vi "NI_9252 DataCollection.vi"(11 "device name":tag="cDAQ9189-21D2231Mod8") -> (3 "First Channel 1D data array":dbl[](array[numeric]))   [LabVIEW 2022 SP3]
uses:
  <vilib>/Analysis/baseanly.llb/Mean (DBL).vi
  STOP_GLOBAL.vi
  <vilib>/Analysis/NI_AALBase.lvlib
panel:
  out "Voltage Chamber Pressure  2":dynamicdata(graph)
  in  "Types of Testing":T1(tab)
  in  "Channel Array":dbl[](array[knob]) scale=0.0..10.0
  in  "maximum voltage":dbl=5.0 format="%0.2f"
  in  "minimum voltage":dbl=-5.0 format="%0.2f"
  in  "Output Channels":tag
  out "Mass Flow":dbl[](graph)
  out "Mass Flow":dynamicdata(graph)
  out "Chamber Pressure":dbl[](graph)
  out "Supply Pressure":dbl[](graph)
  out "Voltage Chamber Pressure":dynamicdata(graph)
  out "Voltage Supply Pressure":dynamicdata(graph)
  # "ANALOG VOLTAGE OUTPUT"
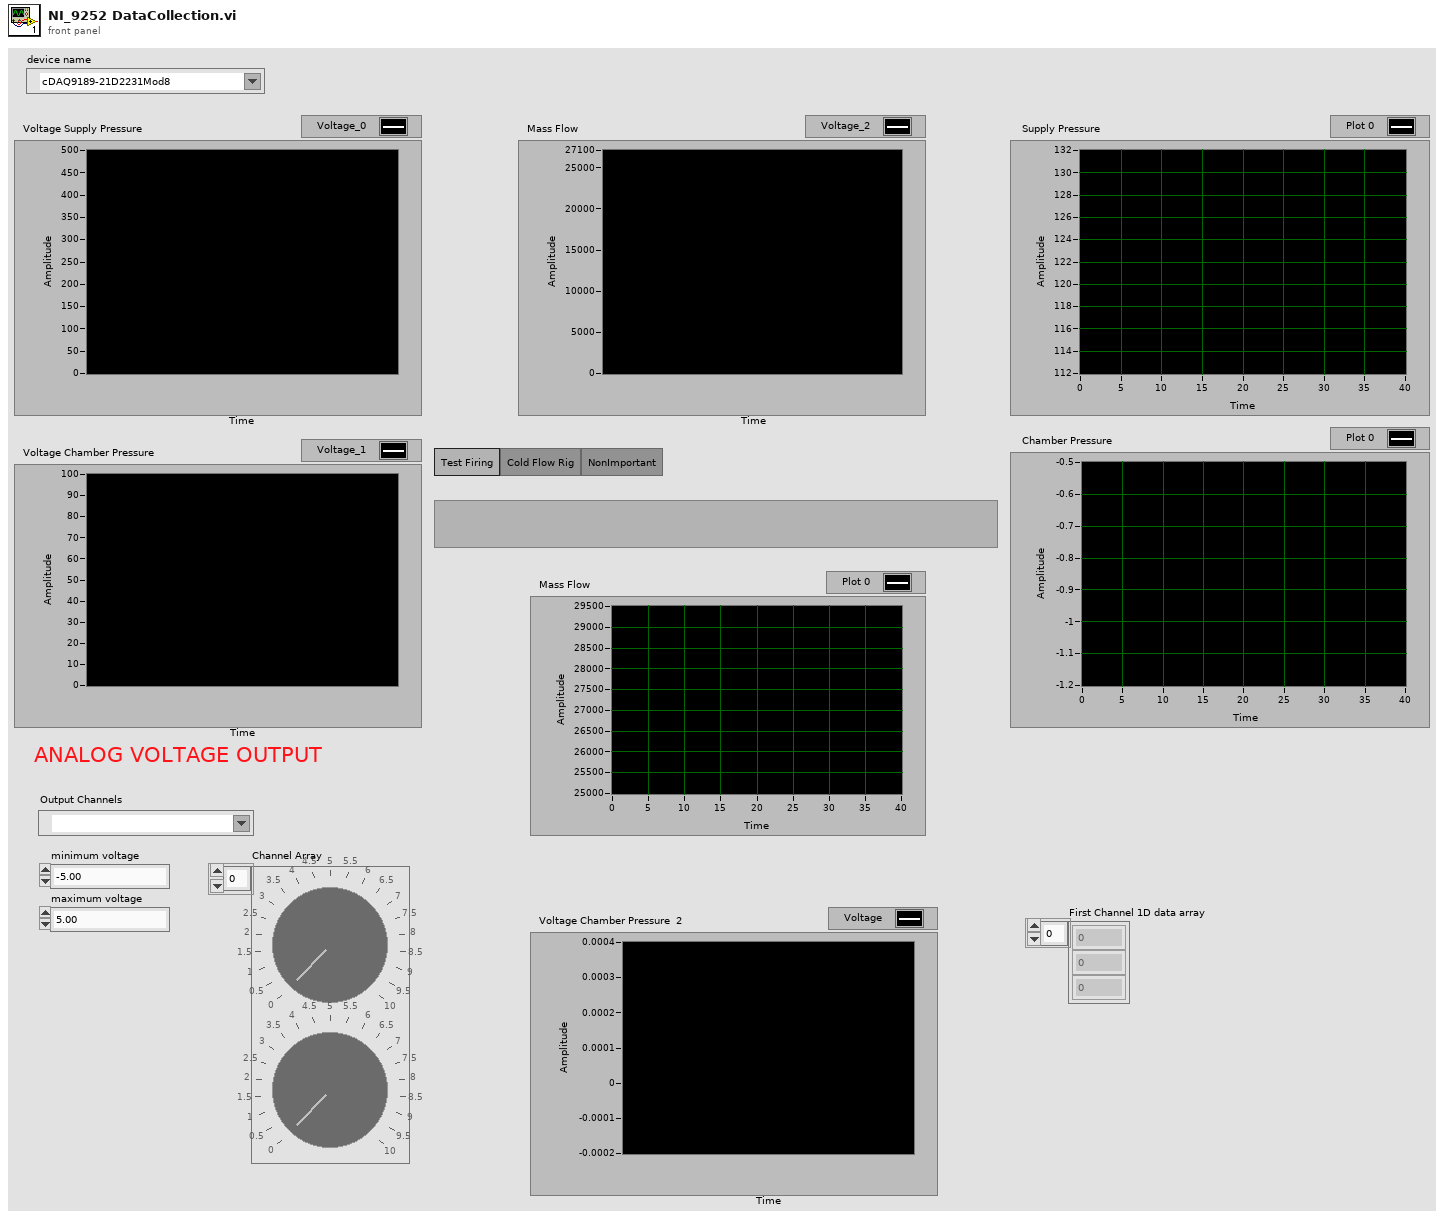
[diagram p1: front panel]
types:
  T1 = enum32{"Test Firing", "Cold Flow Rig", "NonImportant"}
  T2 = enum16{"Left Button", "Center Button", "Right Button", "Window Close"}
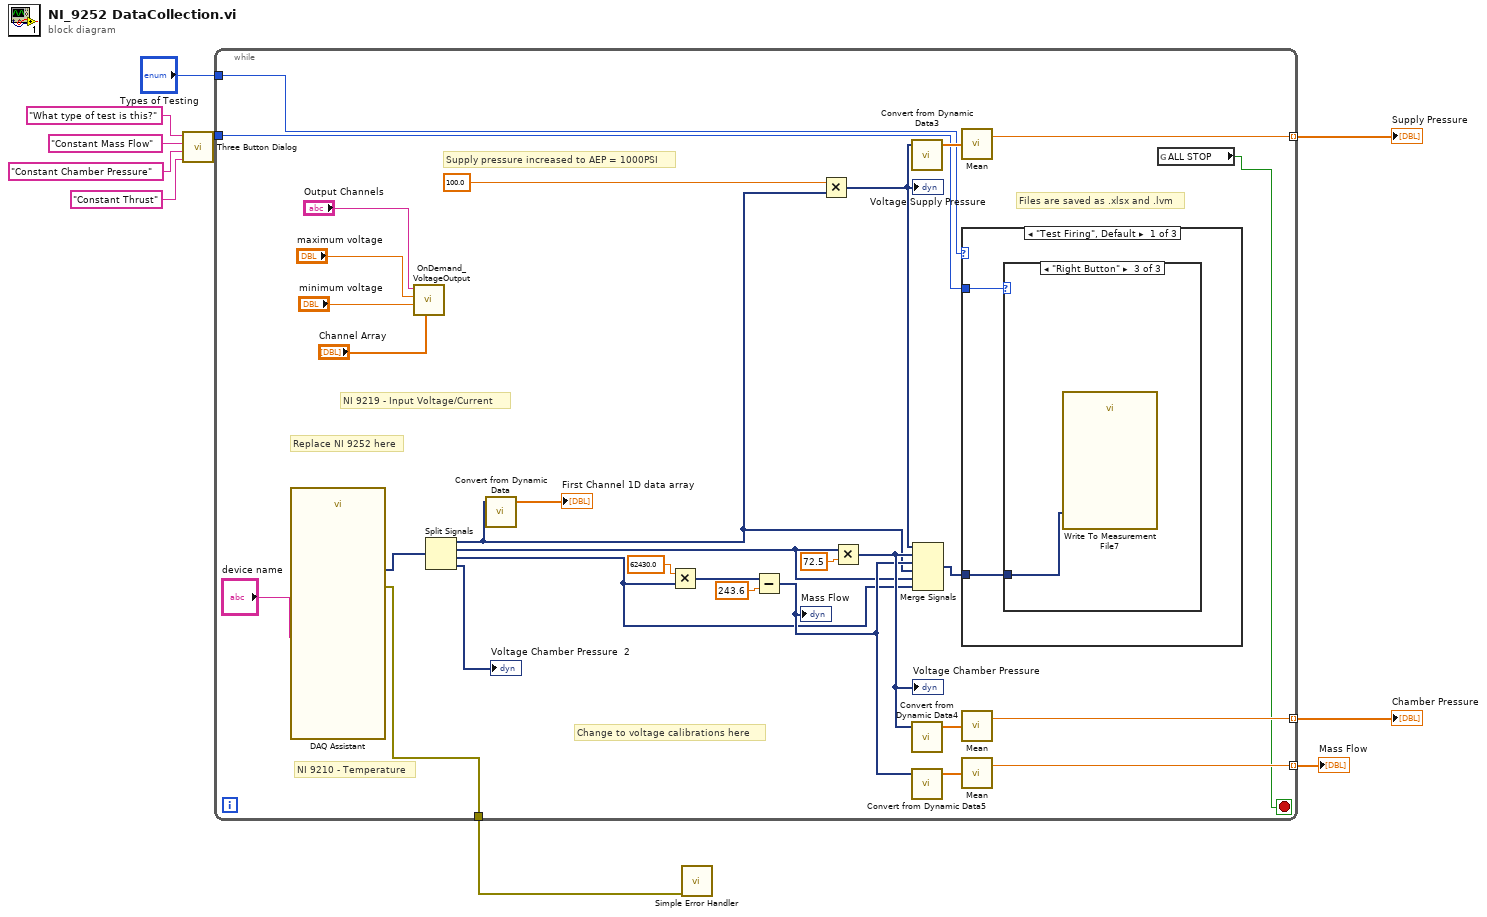
[diagram p0: block diagram]
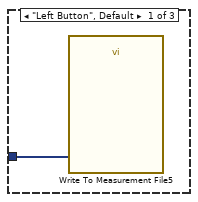
[diagram p2: hidden frame]
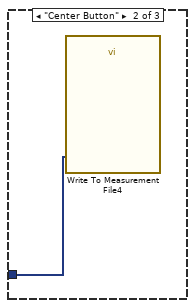
[diagram p3: hidden frame]
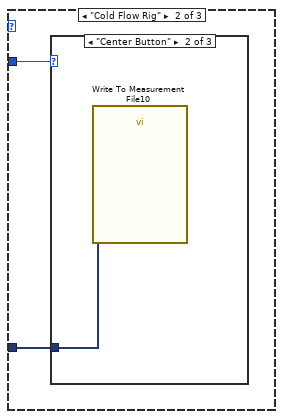
[diagram p4: hidden frame]
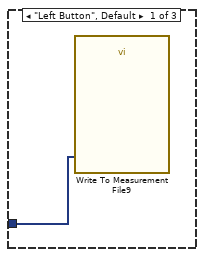
[diagram p5: hidden frame]
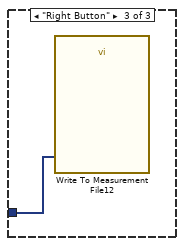
[diagram p6: hidden frame]
diagram:
  n1 = call <vilib>:"Three Button Dialog.vi"("Right Button Text (\"Cancel\")"="Constant Thrust" ("Right Button Text (\"Cancel\")"), "Center Button Text (\"No\")"="Constant Chamber Pressure" ("Center Button Text (\"No\")"), "Left Button Text (\"Yes\")"="Constant Mass Flow" ("Left Button Text (\"Yes\")"), "message"="What type of test is this?") -> ("Which Button?"=w3:T2)  [unwired: 7 in]
  n2 = while {
    tunnel: [w39] -> w10 mode=indexing
    tunnel: [w35] -> w9 mode=indexing
    tunnel: [w30] -> w8 mode=indexing
    tunnel: w3 -> [w21]
    tunnel: "Types of Testing" -> [w22]
    tunnel: [w11] -> w1
    stop <- w17 stop-if-true
    # "Change to voltage calibrations here"
    # "Replace NI 9252 here"
    # "Files are saved as .xlsx and .lvm"
    # "NI 9210 - Temperature"
    # "Supply pressure increased to AEP = 1000PSI"
    # "NI 9219 - Input Voltage/Current"
    n3 = call "DAQ Assistant"("device name"="device name") -> ("data"=w13:dynamicdata, "error out"=w11:errorcluster)  [unwired: 15 in, 2 out]
    n4 = call "OnDemand_VoltageOutput.vi"("Channel Array"="Channel Array", "minimum voltage"="minimum voltage", "maximum voltage"="maximum voltage", "physical channels"="Output Channels") -> ()  [unwired: 7 in, 1 out]
    n5 = Split Signals(w13) -> (w15:dynamicdata, w19:dynamicdata, w18:dynamicdata, →"Voltage Chamber Pressure  2":dynamicdata)  [unwired: 4 in]
    n6 = call "Convert from Dynamic Data"("Dynamic Data Type"=w15) -> ("Array"=→"First Channel 1D data array":dbl[])  [unwired: 3 in]
    n7 = Multiply(x=62430.0, y=w18) -> (x*y=w32:dynamicdata)
    n8 = Subtract(x=w32, y=243.6) -> (x-y=w27:dynamicdata)
    "Mass Flow" <- w27
    n9 = Multiply(x=100.0, y=w15) -> (x*y=w29:dynamicdata)
    "Voltage Supply Pressure" <- w29
    n10 = Multiply(x=w19, y=72.5 ("x")) -> (x*y=w28:dynamicdata)
    "Voltage Chamber Pressure" <- w28
    n11 = call "Convert from Dynamic Data3"("Dynamic Data Type"=w29) -> ("Array"=w31:dbl[])  [unwired: 3 in]
    n12 = call "Convert from Dynamic Data4"("Dynamic Data Type"=w28) -> ("Array"=w40:dbl[])  [unwired: 3 in]
    n13 = call "Convert from Dynamic Data5"("Dynamic Data Type"=w27) -> ("Array"=w36:dbl[])  [unwired: 3 in]
    n14 = Merge Signals(w29, w28, w27, w15, w19, w18) -> (w20:dynamicdata)
    n15 = call-poly <vilib>:"Mean.vi"("X"=w31) -> ("mean"=w30:dbl)  [unwired: 1 out]
    n16 = case shown="\"Test Firing\", Default" w22 {
      tunnel: w21 -> [w42 w47 _]
      tunnel: w20 -> [w41 w46 _]
      frame "Test Firing", Default {
        n17 = case shown="\"Right Button\"" w42 {
          tunnel: w41 -> [w43 w44 w45]
          frame "Left Button", Default {
            n18 = call "Write To Measurement File5"("Signals"=w43) -> ()  [unwired: 16 in, 3 out]
          }
          frame "Center Button" {
            n19 = call "Write To Measurement File4"("Signals"=w44) -> ()  [unwired: 16 in, 3 out]
          }
          frame "Right Button" {
            n20 = call "Write To Measurement File7"("Signals"=w45) -> ()  [unwired: 16 in, 3 out]
          }
        }
      }
      frame "Cold Flow Rig" {
        n21 = case shown="\"Center Button\"" w47 {
          tunnel: w46 -> [w48 w49 w50]
          frame "Left Button", Default {
            n22 = call "Write To Measurement File9"("Signals"=w48) -> ()  [unwired: 16 in, 3 out]
          }
          frame "Center Button" {
            n23 = call "Write To Measurement File10"("Signals"=w49) -> ()  [unwired: 16 in, 3 out]
          }
          frame "Right Button" {
            n24 = call "Write To Measurement File12"("Signals"=w50) -> ()  [unwired: 16 in, 3 out]
          }
        }
      }
      frame "NonImportant" {
      }
    }
    n25 = call-poly <vilib>:"Mean.vi"("X"=w40) -> ("mean"=w39:dbl)  [unwired: 1 out]
    n26 = call-poly <vilib>:"Mean.vi"("X"=w36) -> ("mean"=w35:dbl)  [unwired: 1 out]
    n27 = global read "STOP_GLOBAL.vi" "ALL STOP"() -> (w17:bool)
  }
  "Supply Pressure" <- w8
  "Chamber Pressure" <- w10
  "Mass Flow" <- w9
  n28 = call <vilib>:"Simple Error Handler.vi"("error in (no error)"=w1) -> ()  [unwired: 4 in, 5 out]
